vi "Framework.Rx.vi"(8 "error in (no error)":errorcluster, 11 "Framework in":refnum<class "Framework.lvclass">) -> (0 "error out":errorcluster, 3 "Framework out":refnum<class "Framework.lvclass">)   [LabVIEW 2017, in "DSF Core.lvlib" / "Framework.lvclass"]
uses:
  Framework.lvclass
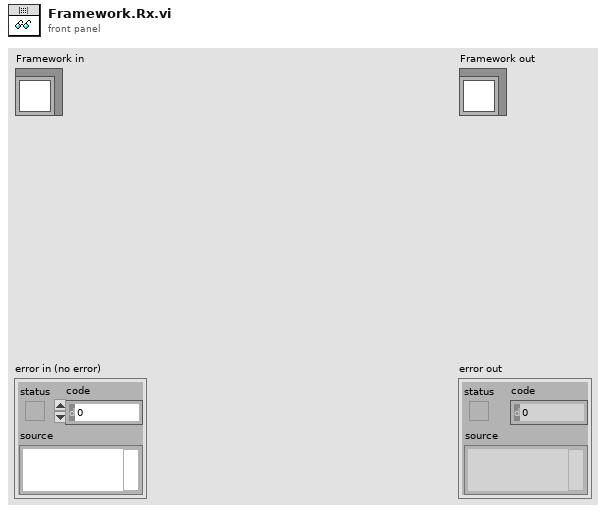
[diagram p1: front panel]
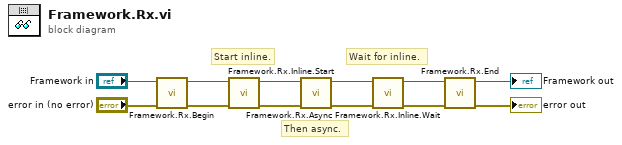
[diagram p0: block diagram]
diagram:
  # "Wait for inline."
  # "Start inline."
  # "Then async."
  n1 = call "Framework.Rx.Begin.vi"("error in (no error)"="error in (no error)", "Framework in"="Framework in") -> ("error out"=w9:errorcluster, "Framework out"=w10:refnum<class "Framework.lvclass">)  [unwired: 8 in]
  n2 = call "Framework.Rx.Inline.Start.vi"("error in (no error)"=w9, "Framework in"=w10) -> ("error out"=w1:errorcluster, "Framework out"=w2:refnum<class "Framework.lvclass">)  [unwired: 8 in]
  n3 = call "Framework.Rx.Async.vi"("error in (no error)"=w1, "Framework in"=w2) -> ("error out"=w4:errorcluster, "Framework out"=w3:refnum<class "Framework.lvclass">)  [unwired: 8 in]
  n4 = call "Framework.Rx.Inline.Wait.vi"("error in (no error)"=w4, "Framework in"=w3) -> ("error out"=w8:errorcluster, "Framework out"=w7:refnum<class "Framework.lvclass">)  [unwired: 8 in]
  n5 = call "Framework.Rx.End.vi"("error in (no error)"=w8, "Framework in"=w7) -> ("error out"=→"error out":errorcluster, "Framework out"=→"Framework out":refnum<class "Framework.lvclass">)  [unwired: 8 in]
